vi "Area.vi"(11 "Numeric in":dbl) -> (3 "Numeric out":dbl)   [LabVIEW 2018]
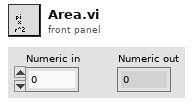
[diagram p1: front panel]
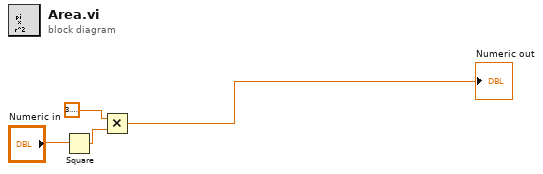
[diagram p0: block diagram]
diagram:
  n1 = Square(x="Numeric in") -> (x^2=w3:dbl)
  n2 = Multiply(x=3.141592653589793, y=w3) -> (x*y=→"Numeric out":dbl)
